vi "cm_Channel Monitor Init.vi"(3 "Container State":T4, 4 "Previous State":variant, 5 "Previous Version":T3) -> (2 "Current State":T1={"Chan"=[], "First Drop?"=FALSE, "Notifier Name"="", "Refresh View"=FALSE, "Scale to Input Range"=FALSE, "Linear View"=FALSE, "Display"={"Current"=6618880, "Peak"=6618880}, "Property/Method"=enum."No Update", "Time Display Ref"=[]})   [LabVIEW 2009, in "Channel Monitor [System].xctl"]
uses:
  Channel Monitor [System].xctl
  cm_Channel Monitor State.ctl
  TypeDef/cm_Property_Method.ctl
  <vilib>/_xctls/Container State.ctl
  <vilib>/_xctls/Version.ctl
  cm_XControlState Action.ctl
  <vilib>/_xctls/XControlSupport.lvlib
panel:
  in  "Default Indicator State":T1={"Chan"=[], "First Drop?"=TRUE, "Notifier Name"="", "Refresh View"=FALSE, "Scale to Input Range"=FALSE, "Linear View"=TRUE, "Display"={"Current"=16860, "Peak"=16711680}, "Property/Method"=enum."No Update", "Time Display Ref"=[]}
  in  "Default Control State":T1={"Chan"=[], "First Drop?"=TRUE, "Notifier Name"="", "Refresh View"=FALSE, "Scale to Input Range"=FALSE, "Linear View"=TRUE, "Display"={"Current"=16860, "Peak"=16711680}, "Property/Method"=enum."No Update", "Time Display Ref"=[]}
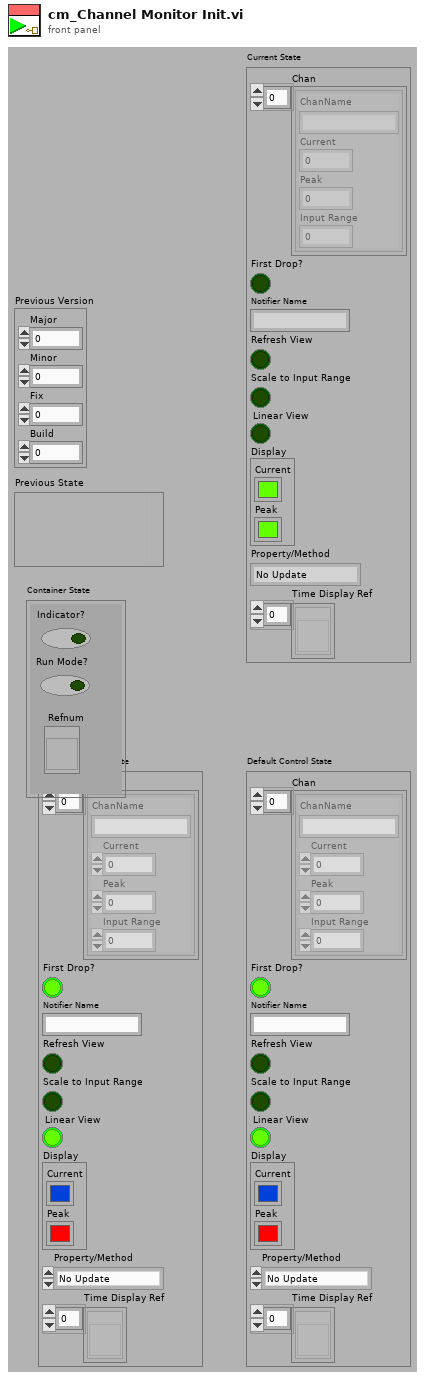
[diagram p1: front panel]
types:
  T1 = typedef "Channel Monitor [System].xctl/cm_Channel Monitor State.ctl" = cluster{"Chan":cluster{"ChanName":string, "Current":dbl, "Peak":dbl, "Input Range":dbl}[], "First Drop?":bool, "Notifier Name":string, "Refresh View":bool, "Scale to Input Range":bool, "Linear View":bool, "Display":cluster{"Current":u32, "Peak":u32}, "Property/Method":T2, "Time Display Ref":refnum<vi>[]}
  T2 = typedef "Channel Monitor [System].xctl/cm_Property_Method.ctl" = enum16{"No Update", "Color: Currrent", "Color: Peak", "Close Time Displays"}
  T3 = typedef "XControlSupport.lvlib/Version.ctl" = cluster{"Major":u16, "Minor":u16, "Fix":u16, "Build":u16}
  T4 = typedef "XControlSupport.lvlib/Container State.ctl" = cluster{"Indicator?":bool, "Run Mode?":bool, " Refnum":refnum<vi>}
  T5 = typedef "Channel Monitor [System].xctl/cm_XControlState Action.ctl" = enum16{"Add", "Write", "Read", "Remove"}
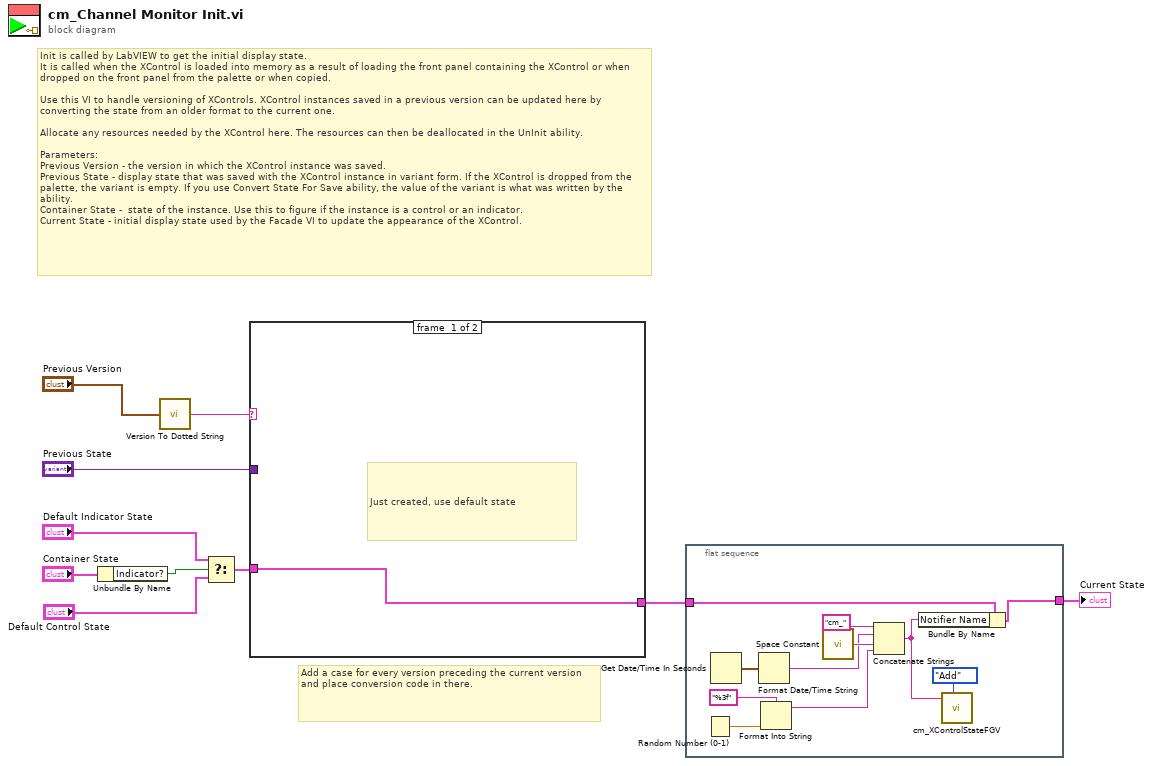
[diagram p0: block diagram]
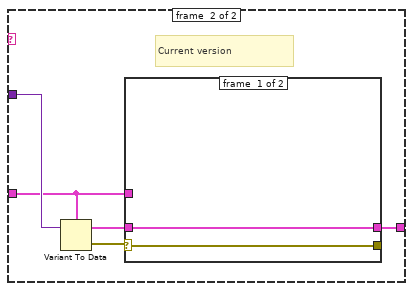
[diagram p2: hidden frame]
diagram:
  # "Add a case for every version preceding the current version and place conversion code in there."
  # "Init is called by LabVIEW to get the initial display state.\nIt is called when the XControl is loaded into memory as a result of loading the front panel containing the XControl or when dropped on the front panel from the palette or when copied.\n\nUse this VI to handle versioning of XControls. XControl instances saved in a previous version can be updated here by converting the state from an older format to the current one.\n\nAllocate any resources needed by the XControl here. The resources can then be deallocated in the UnInit ability.\n\nParameters:\nPrevious Version - the version in which the XControl instance was saved.\nPrevious State - display state that was saved with the XControl instance in variant form. If the XControl is dropped from the palette, the variant is empty. If you use Convert State For Save ability, the value of the variant is what was written by the ability. \nContainer State -  state of the instance. Use this to figure if the instance is a control or an indicator.\nCurrent State - initial display state used by the Facade VI to update the appearance of the XControl."
  n1 = Unbundle By Name("Container State") -> ("Indicator?"=w6:bool)
  n2 = call <vilib>:"Version To Dotted String.vi"("Version"="Previous Version") -> ("String Version"=w1:string)
  n3 = Select(t="Default Indicator State", s=w6, f="Default Control State") -> (s? t:f=w5:T1)
  n4 = case shown="\"\", Default" w1 {
    tunnel: "Previous State" -> [_ w16]
    tunnel: [w11 w12] -> w3
    tunnel: w5 -> [w11 w13]
    frame #0 {
      # "Just created, use default state"
    }
    frame #1 {
      # "Current version"
      n5 = Variant To Data(Variant=w16, type=w13) -> (error out=w15:errorcluster, data=w14:T1)  [unwired: 1 in]
      n6 = case shown="No Error" w15 {
        selector: w15 -> [w18 w19]
        tunnel: w14 -> [w17 _]
        tunnel: [w17 w20] -> w12
        tunnel: w13 -> [_ w20]
        tunnel: [w18 w19] -> _
        frame #0 {
        }
        frame #1 {
          # "Error converting previously \nsaved state. Use default instead."
        }
      }
    }
  }
  n7 = flat-sequence {
    tunnel: w3 -> [w30]
    tunnel: [w29] -> w4
    frame #0 {
      n8 = Random Number (0-1)() -> (number: 0 to 1=w24:dbl)
      n9 = Get Date/Time In Seconds() -> (seconds since 1Jan1904=w27:timestamp)
      n10 = Format Date/Time String(seconds (now)=w27) -> (date/time string=w25:string)  [unwired: 2 in]
      n11 = Format Into String(format string="%3f", w24) -> (resulting string=w23:string)  [unwired: 2 in, 1 out]
      n12 = call <vilib>:"Space Constant.vi"() -> ("String"=w26:string)
      n13 = Concatenate Strings("cm_", w25, w26, w23) -> (w21:string)
      n14 = Bundle By Name(cluster=w30, "Notifier Name"=w21) -> (w29:T1)
      n15 = call "cm_XControlStateFGV.vi"("Action"=cm_XControlState_Action."Add", "XControl Name"=w21) -> ()  [unwired: 6 in, 4 out]
    }
  }
  "Current State" <- w4
